vi "STAGE+mono+counter_edit-3x-error.vi"() -> ()   [LabVIEW 2017]
panel:
  out "XY Graph":cluster{"Y":dbl[], "Y":dbl[]}[](graph)
  in  "Integrating time, 10^-7 sec":dbl=10000000.0
  in  "scan from":i32=2600
  in  "scan to":i32=4000
  in  "?":bool
  in  "Exit Labview":bool
  in  "step size":dbl=10.0 min=0.0
  in  "?":bool
  out "Spectrum":waveform(dbl)(graph)
  out "Counts":i32
  in  "value (0)":dbl=-9.0
  in  "number of disc steps":i32=1
  out "Current WL Wavelength  2":u16 caption="Current Wavelength"
  out "Grt# 2":u8=1 min=1 max=3 step=1
  out "Blaze (nm)":u32=300
  out "Groove/mm":u32=1200
  in  "?":bool
  in  "Channel B Input":u16(ring)=2 items=["Input 1"=1, "Input 2"=2]
  in  "Trigger mode":u16(ring) items=["10 MHz"=0, "Input 2"=2, "Input T"=3]
  out "Current WL Wavelength":u16 caption="Current Wavelength"
  in  "Integrating time, 10^-7 sec":dbl=10000000.0
  in  "gate A mode (CW:0)":i16(slide) scale=0.0..2.0 scale format="%.2f"
  in  "Channel A Input":u16(ring)=1 items=["10 MHz", "Input 1"]
  in  "Time between measurements\n at one point (s)/Dwell Time":dbl=0.002 min=0.002 max=60.0 step=0.001
  in  "Number of Measurements\n to take at one point/ Number of Periods":u16=1 min=1 max=2000 step=1
  in  "Count Mode":u16(ring) items=["A,B for Preset T", "A-B for Preset T", "A+B for Preset T", "A for Preset B"]
  in  "GPIB address":string="23"
  out "Timeout":bool
  out "Serial":u32=12345
  out "Grt#":u8=1 min=1 max=3 step=1
  out "Blaze (nm)":u32=300
  out "Groove/mm":u32=1200
  out "time delay":u32=450000 min=1
  out "Mono port":T1(ring)
  in  "Get position":bool
  out "Position status":dbl format="%.3f"
  in  "Target position":dbl format="%.3f"
  in  "Move":bool
  in  "Motor OFF":bool
  in  "Motor ON":bool
  in  "Step Size [um]":i32=10
  in  "Axis":i32=1
  in  "Rep Rate [Hz]":dbl=500.0
  out "Shots":dbl
  in  "Averaging Time [s]":dbl=0.1
  out "Current Point":i32
  out "Slide":i32(slide) scale=0.0..100.0
  out "Current Position [mm]":dbl
  in  "Axis initial position [mm]":dbl
  out "Axis final Position [mm]":dbl
  in  "Data Points (100 default)":i32=100
  in  "Collect Data!":bool
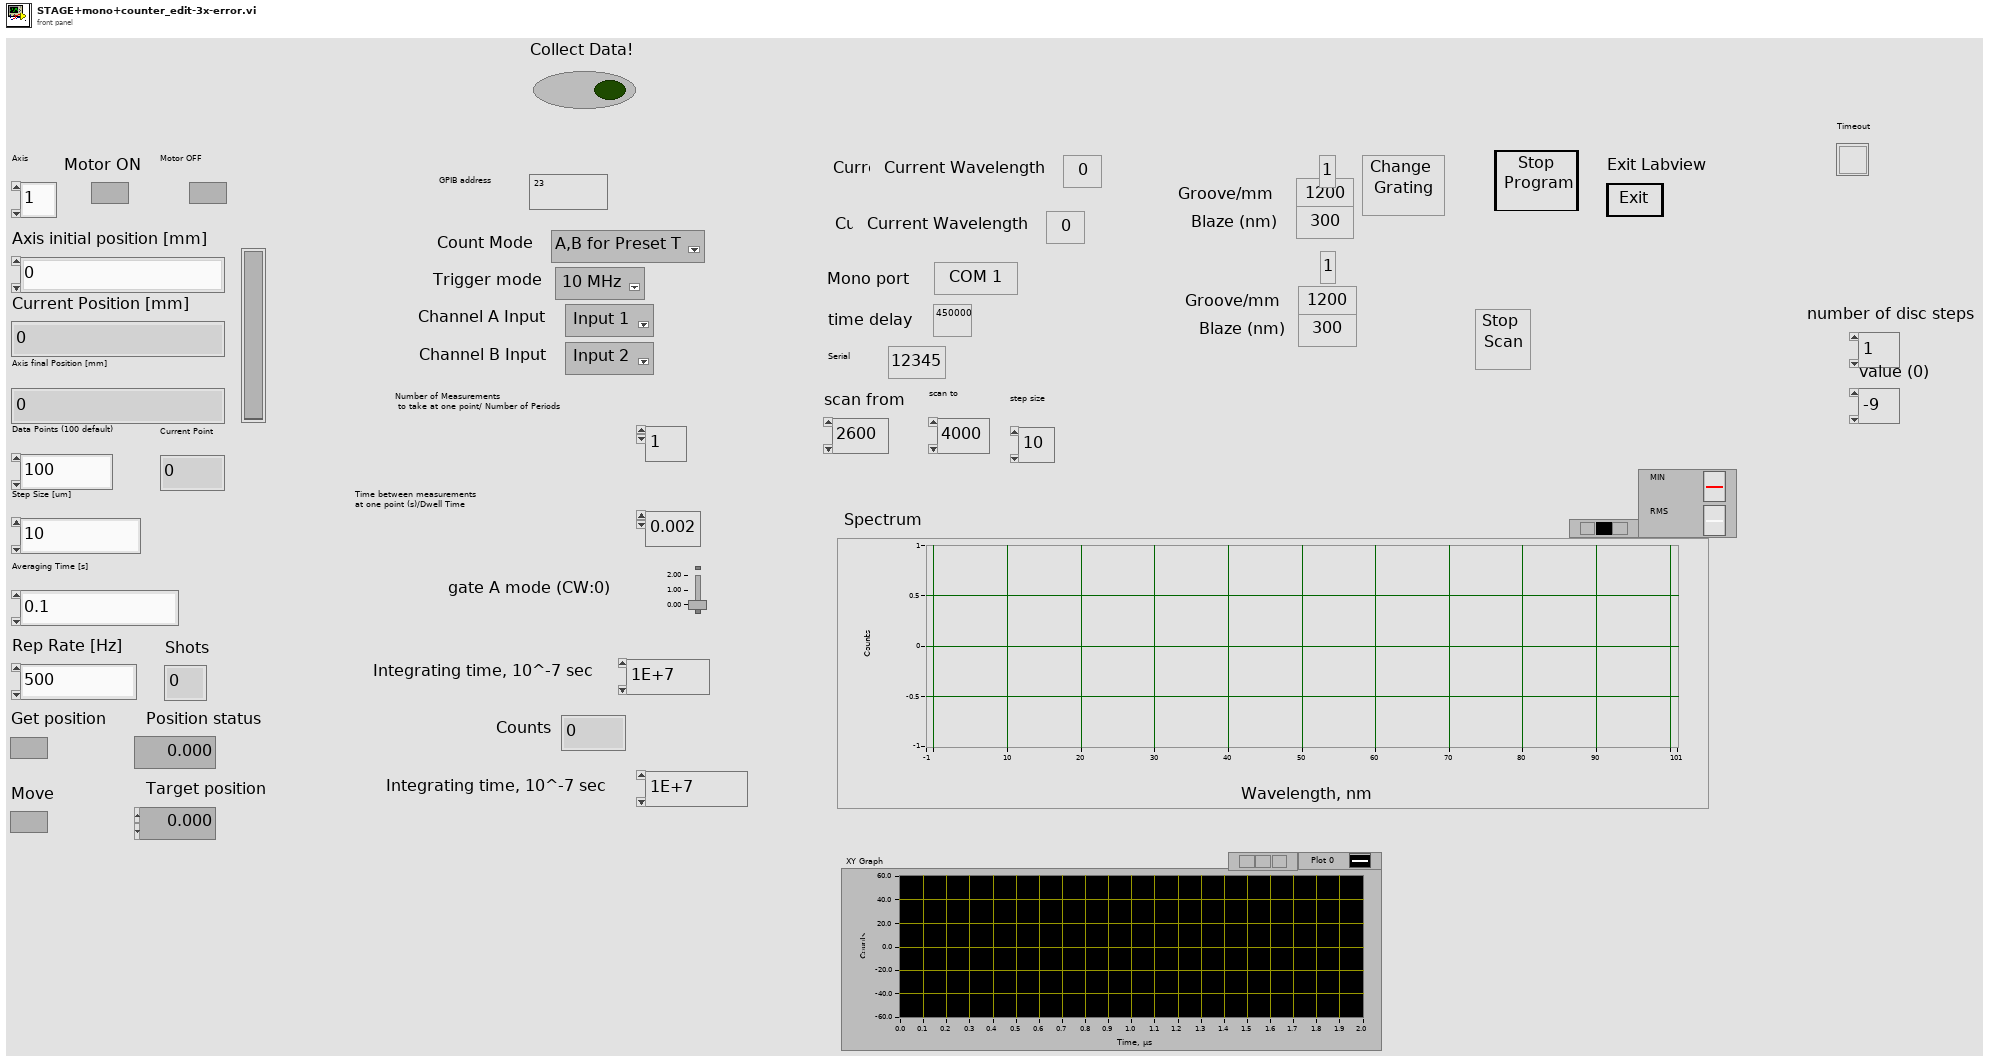
[diagram p1: front panel]
types:
  T1 = enum8{"COM 1", "COM 2", "COM 3", "COM 4", "COM 5", "COM 6", "COM 7", "COM 8", "COM 9"}
  T2 = cluster{"input XON/XOFF":bool, "input HW Handshake":bool, "input alt HW HShk":bool, "output XON/XOFF":bool, "output HW Handshake":bool, "output alt HW HShk":bool, "XOFF byte":u8, "XON byte":u8, "parity error byte":u16}
  T3 = enum16{"no parity", "odd parity", "even parity", "mark parity", "space parity"}
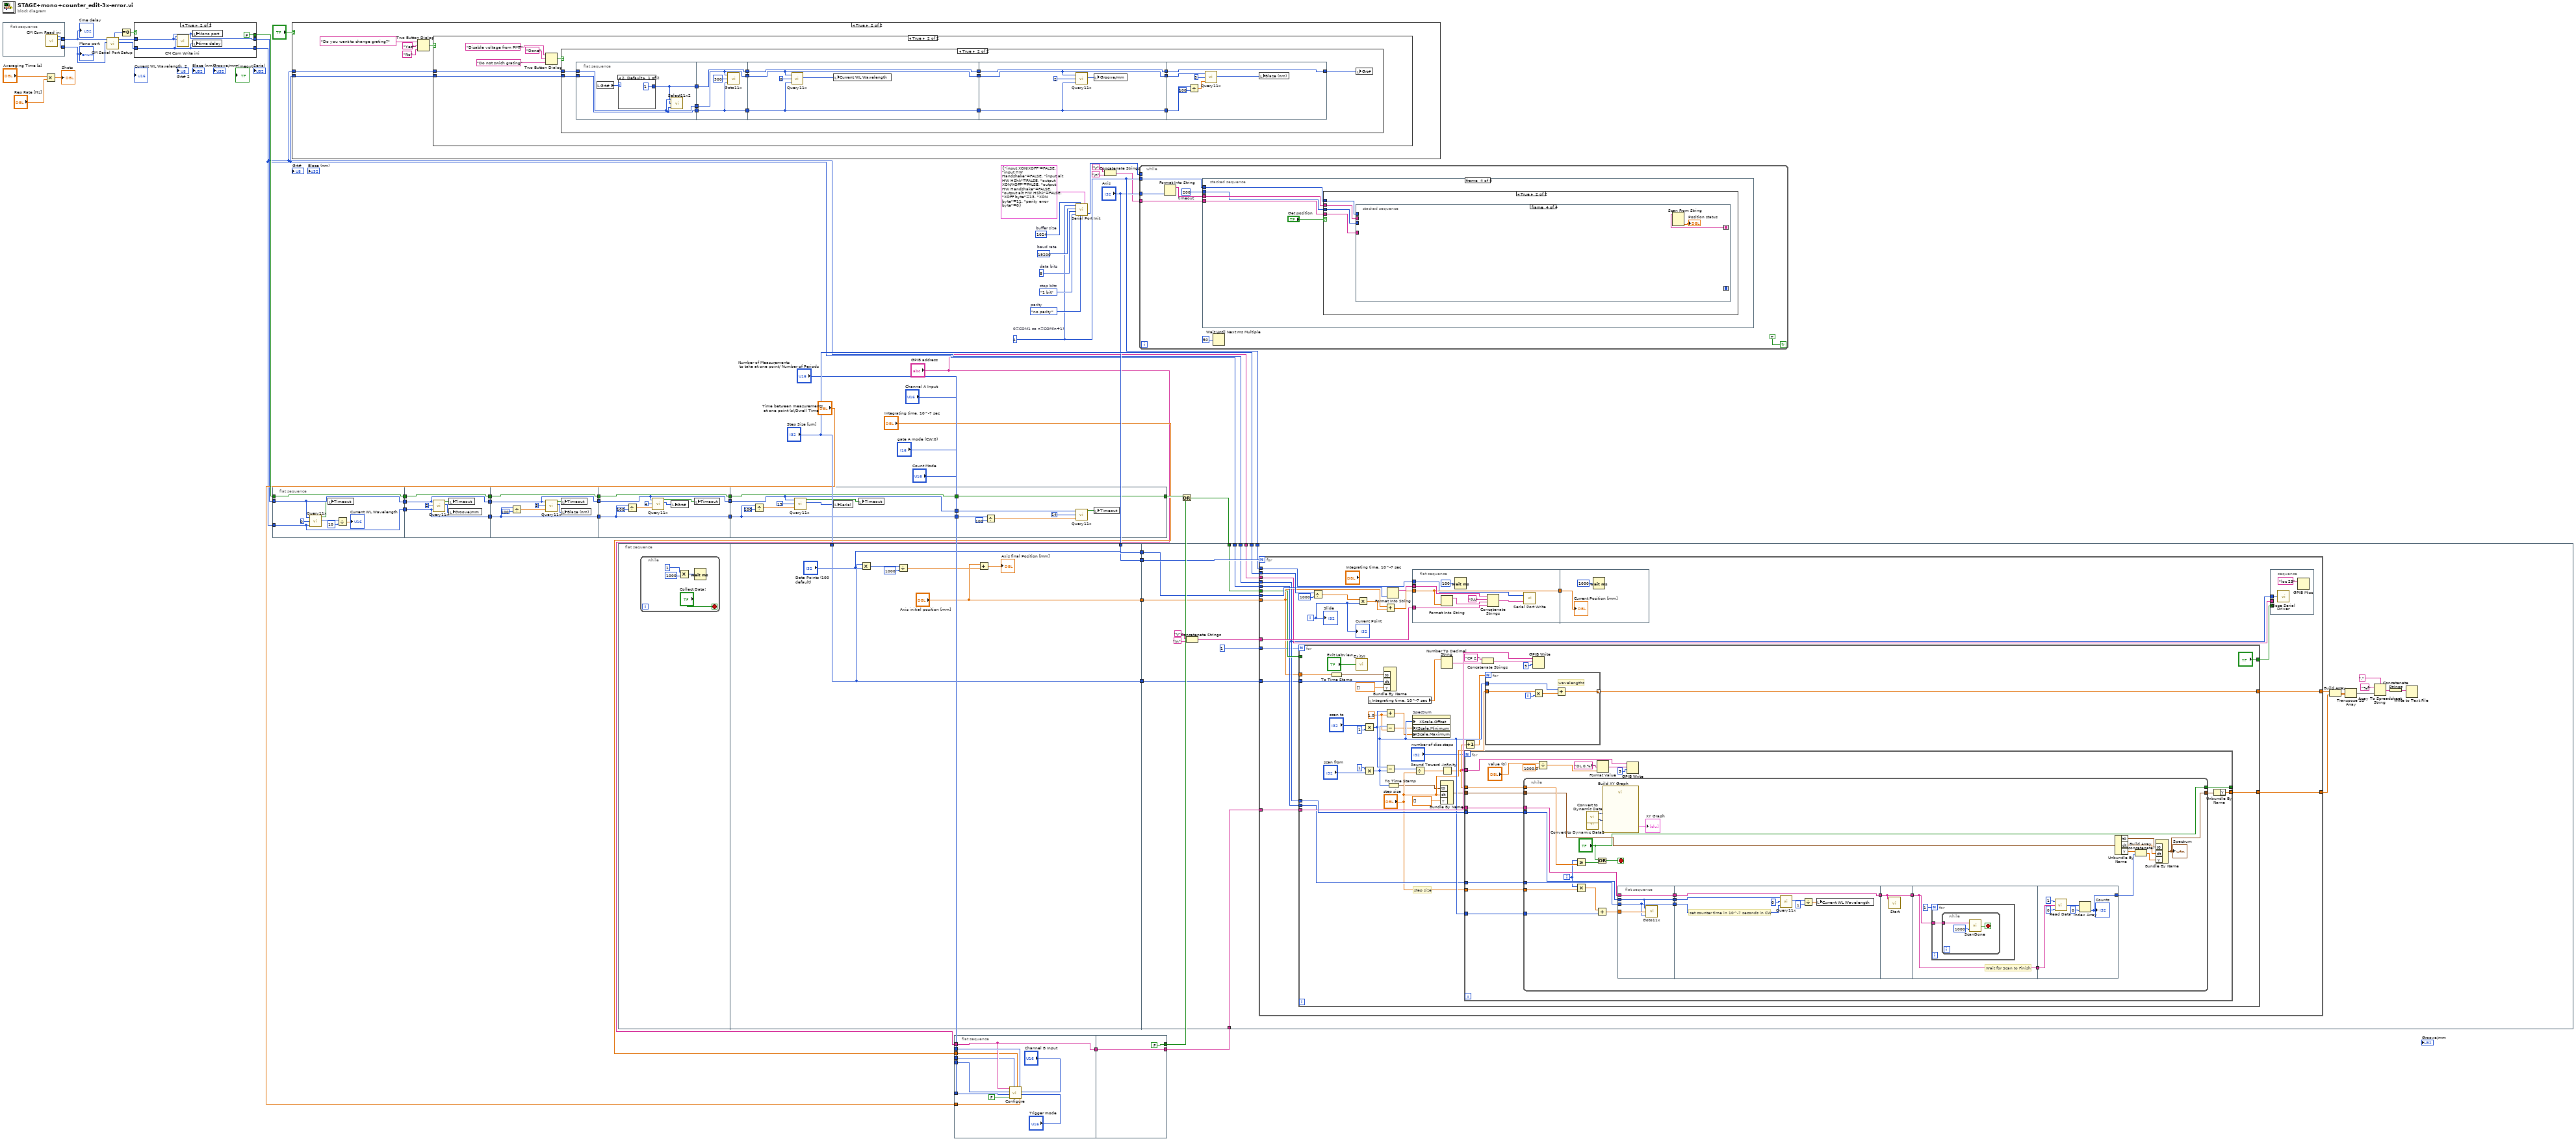
[diagram p0: block diagram]
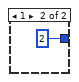
[diagram p5: hidden frame]
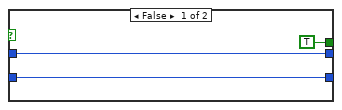
[diagram p6: hidden frame]
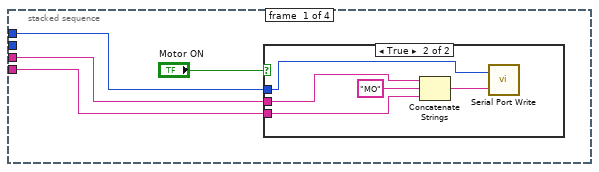
[diagram p7: hidden frame]
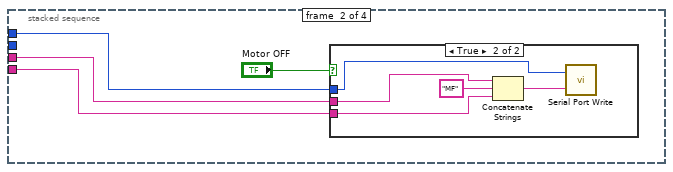
[diagram p9: hidden frame]
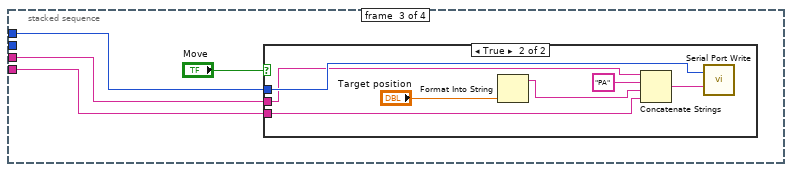
[diagram p11: hidden frame]
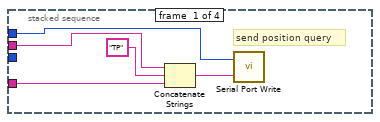
[diagram p14: hidden frame]
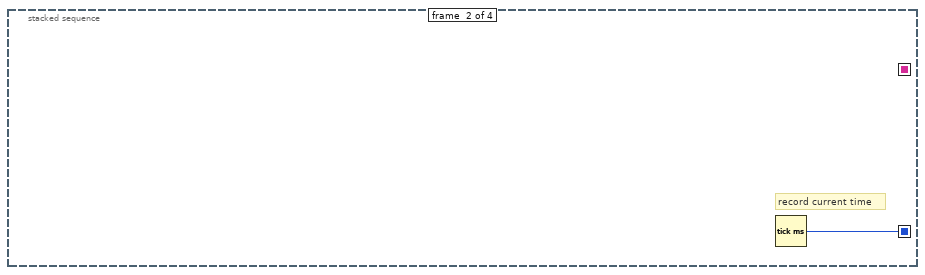
[diagram p15: hidden frame]
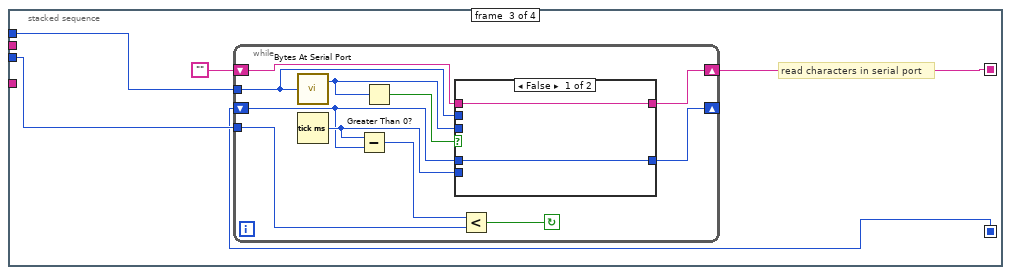
[diagram p16: hidden frame]
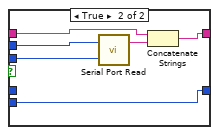
[diagram p17: hidden frame]
diagram:
  w47 = u32 19200  # baud rate
  w46 = u16 8  # data bits
  w45 = enum16{"1 bit", "1.5 bits", "2 bits"}."1 bit"  # stop bits
  w50 = T3."no parity"  # parity
  w44 = 4  # 0=COM1 so n=COM(n+1)
  w49 = u16 1024  # buffer size
  n1 = flat-sequence {
    tunnel: [w59] -> w22
    tunnel: [w58] -> w21
    frame #0 {
      n2 = call "CM Com Read ini.vi"() -> ("Mono port"=w58:T1, "time delay1"=w59:u32)  [unwired: 7 in]
    }
  }
  n3 = Multiply(x="Averaging Time [s]", y="Rep Rate [Hz]") -> (x*y=→"Shots":dbl)
  n4 = call "CM Serial Port Setup.vi"("COM port"=w21, "time delay"=w22) -> ("time delay1"=w17:u32, "DK port Out"=w18:T1, "error code"=w20:i32)  [unwired: 7 in]
  n5 = Equal To 0?(x=w20) -> (x = 0?=w19:bool)
  n6 = case shown="True" w19 {
    tunnel: w18 -> [w62 w65]
    tunnel: w17 -> [w61 w64]
    tunnel: [w62 w65] -> w4
    tunnel: [w61 w64] -> w3
    tunnel: [TRUE FALSE] -> w16
    frame False {
    }
    frame True {
      n7 = call "CM Com Write ini.vi"("time delay1"=w65, "Mono port"=w64) -> ()  [unwired: 7 in]
      n8 = local write "Mono port"(w65) -> ()
      n9 = local write "time delay"(w64) -> ()
    }
  }
  n10 = flat-sequence {
    tunnel: w3 -> [w71]
    tunnel: [w71] -> w38
    tunnel: w4 -> [w73]
    tunnel: [w73] -> w37
    tunnel: w16 -> [w69]
    tunnel: [w69] -> w36
    tunnel: w38 -> [w76]
    tunnel: [w76] -> w35
    tunnel: w37 -> [w78]
    tunnel: [w78] -> w34
    tunnel: w36 -> [w74]
    tunnel: [w74] -> w33
    tunnel: w35 -> [w86]
    tunnel: [w86] -> w32
    tunnel: w34 -> [w83]
    tunnel: [w83] -> w31
    tunnel: w33 -> [w80]
    tunnel: [w80] -> w30
    tunnel: w32 -> [w94]
    tunnel: [w94] -> w29
    tunnel: w31 -> [w91]
    tunnel: [w91] -> w28
    tunnel: w30 -> [w88]
    tunnel: [w88] -> w27
    tunnel: w29 -> [w102]
    tunnel: [w102] -> w26
    tunnel: w28 -> [w99]
    tunnel: [w99] -> w25
    tunnel: w27 -> [w96]
    tunnel: [w96] -> w24
    tunnel: w26 -> [w109]
    tunnel: w25 -> [w106]
    tunnel: [w104] -> w10
    tunnel: w24 -> [w104]
    frame #0 {
      n11 = call "Query11x.vi"("port number"=w73, "QUERY"=u16 0, "time delay"=w71) -> ("timeout"=w70:bool, "STATUS MESSAGE"=w68:u16)  [unwired: 2 out]
      n12 = local write "Timeout"(w70) -> ()
      n13 = Divide(x=w68, y=10 ("Numeric")) -> (x/y=→"Current WL Wavelength":dbl)
    }
    frame #1 {
      n14 = call "Query11x.vi"("port number"=w78, "QUERY"=u16 2, "time delay"=w76) -> ("timeout"=w75:bool, "STATUS MESSAGE"=w77:u16)  [unwired: 2 out]
      n15 = local write "Timeout"(w75) -> ()
      n16 = local write "Groove/mm"(w77) -> ()
    }
    frame #2 {
      n17 = Divide(x=w86, y=i16 100 ("device (1)")) -> (x/y=w84:dbl)
      n18 = call "Query11x.vi"("port number"=w83, "QUERY"=u16 3, "time delay"=w84) -> ("timeout"=w81:bool, "STATUS MESSAGE"=w82:u16)  [unwired: 2 out]
      n19 = local write "Timeout"(w81) -> ()
      n20 = local write "Blaze (nm)"(w82) -> ()
    }
    frame #3 {
      n21 = Divide(x=w94, y=i16 100 ("device (1)")) -> (x/y=w92:dbl)
      n22 = call "Query11x.vi"("port number"=w91, "QUERY"=u16 4, "time delay"=w92) -> ("timeout"=w89:bool, "STATUS MESSAGE"=w90:u16)  [unwired: 2 out]
      n23 = local write "Grt#"(w90) -> ()
      n24 = local write "Timeout"(w89) -> ()
    }
    frame #4 {
      n25 = Divide(x=w102, y=i16 100 ("device (1)")) -> (x/y=w100:dbl)
      n26 = call "Query11x.vi"("port number"=w99, "QUERY"=u16 19, "time delay"=w100) -> ("timeout"=w97:bool, "STATUS MESSAGE"=w98:u16)  [unwired: 2 out]
      n27 = local write "Serial"(w98) -> ()
      n28 = local write "Timeout"(w97) -> ()
    }
    frame #5 {
      n29 = Divide(x=w109, y=i16 100 ("device (1)")) -> (x/y=w107:dbl)
      n30 = call "Query11x.vi"("port number"=w106, "QUERY"=u16 14, "time delay"=w107) -> ("timeout"=w105:bool)  [unwired: 3 out]
      n31 = local write "Timeout"(w105) -> ()
    }
  }
  n32 = case shown="True" "?" {
    tunnel: w3 -> [_ w112]
    tunnel: w4 -> [_ w111]
    frame False {
    }
    frame True {
      n33 = Two Button Dialog(message="Do you want to change grating?", 1:"No" ("F button name (\"Cancel\")"), 2:"Yes" ("T button name (\"OK\")")) -> (T button?=w113:bool)
      n34 = case shown="True" w113 {
        tunnel: w112 -> [_ w118]
        tunnel: w111 -> [_ w117]
        frame False {
        }
        frame True {
          n35 = Two Button Dialog(message="Disable voltage from PMT", 1:"Do not swich grating" ("F button name (\"Cancel\")"), 2:"Done" ("T button name (\"OK\")")) -> (T button?=w119:bool)
          n36 = case shown="True" w119 {
            tunnel: w118 -> [_ w137]
            tunnel: w117 -> [_ w136]
            frame False {
            }
            frame True {
              n37 = flat-sequence {
                tunnel: w137 -> [w141]
                tunnel: [w141] -> w134
                tunnel: w136 -> [w140]
                tunnel: [w140] -> w133
                tunnel: [w138] -> w132
                tunnel: w134 -> [w145]
                tunnel: [w145] -> w131
                tunnel: w133 -> [w146]
                tunnel: [w146] -> w130
                tunnel: w132 -> [w144]
                tunnel: [w144] -> w129
                tunnel: w131 -> [w152]
                tunnel: [w152] -> w128
                tunnel: w130 -> [w151]
                tunnel: [w151] -> w127
                tunnel: w129 -> [w148]
                tunnel: [w148] -> w126
                tunnel: w128 -> [w155]
                tunnel: [w155] -> w125
                tunnel: w127 -> [w156]
                tunnel: [w156] -> w124
                tunnel: w126 -> [w153]
                tunnel: [w153] -> w123
                tunnel: w125 -> [w160]
                tunnel: w124 -> [w161]
                tunnel: [w158] -> w135
                tunnel: w123 -> [w158]
                frame #0 {
                  n38 = local read "Grt#"() -> (w139:u8)
                  n39 = case shown="2, Default" w139 {
                    tunnel: [1 2] -> w138
                    frame 2, Default {
                    }
                    frame 1 {
                    }
                  }
                  n40 = call "Select11x2.vi"("time delay"=w141, "NEW GRT?"=w138, "port number"=w140) -> ()  [unwired: 3 out]
                }
                frame #1 {
                  n41 = call "Goto11x.vi"("time delay"=w145, "WAVELENGTH"=u16 300, "port number"=w146) -> ()  [unwired: 3 out]
                }
                frame #2 {
                  n42 = call "Query11x.vi"("port number"=w151, "QUERY"=u16 0, "time delay"=w152) -> ("STATUS MESSAGE"=w149:u16)  [unwired: 3 out]
                  n43 = local write "Current WL Wavelength"(w149) -> ()
                }
                frame #3 {
                  n44 = call "Query11x.vi"("port number"=w156, "QUERY"=u16 2, "time delay"=w155) -> ("STATUS MESSAGE"=w154:u16)  [unwired: 3 out]
                  n45 = local write "Groove/mm"(w154) -> ()
                }
                frame #4 {
                  n46 = Divide(x=w160, y=i16 100 ("device (1)")) -> (x/y=w162:dbl)
                  n47 = call "Query11x.vi"("port number"=w161, "QUERY"=u16 3, "time delay"=w162) -> ("STATUS MESSAGE"=w159:u16)  [unwired: 3 out]
                  n48 = local write "Blaze (nm)"(w159) -> ()
                }
              }
              n49 = local write "Grt#"(w135) -> ()
            }
          }
        }
      }
    }
  }
  n50 = flat-sequence {
    tunnel: ["Data Points (100 default)"] -> w57
    tunnel: "Axis" -> [w176]
    tunnel: ["Axis initial position [mm]"] -> w56
    tunnel: "Step Size [um]" -> [w169]
    tunnel: [w176] -> w55
    tunnel: [w169] -> w1
    tunnel: w57 -> [w199]
    tunnel: w56 -> [w198]
    tunnel: "Step Size [um]" -> [w197]
    tunnel: w55 -> [w196]
    tunnel: w44 -> [w192]
    tunnel: w6 -> [w191]
    tunnel: w5 -> [w190]
    tunnel: w4 -> [w189]
    tunnel: w3 -> [w188]
    tunnel: "GPIB address" -> [w187]
    tunnel: w1 -> [w185]
    frame #0 {
      n51 = while {
        stop <- "Collect Data!" stop-if-true
        n52 = Multiply(x=1, y=1000) -> (x*y=w168:i32)
        n53 = Wait (ms)(milliseconds to wait=w168) -> ()  [unwired: 1 out]
      }
    }
    frame #1 {
      n54 = Multiply(x=w169, y="Data Points (100 default)") -> (x*y=w172:i32)
      n55 = Divide(x=w172, y=1000) -> (x/y=w171:dbl)
      n56 = Add(x="Axis initial position [mm]", y=w171) -> (x+y=→"Axis final Position [mm]":dbl)
    }
    frame #2 {
      n57 = Concatenate Strings("\r", "\n") -> (w193:string)
      n58 = for {
        N: w199 -> [_]
        tunnel: w198 -> [w203]
        tunnel: w197 -> [w217]
        tunnel: w196 -> [w214]
        tunnel: w193 -> [w211]
        tunnel: w192 -> [w212]
        tunnel: w191 -> [w209]
        tunnel: w190 -> [w208]
        tunnel: w189 -> [w205]
        tunnel: w188 -> [w207]
        tunnel: w187 -> [w206]
        tunnel: 1 -> [w204]
        tunnel: w185 -> [w202]
        tunnel: [w201] -> w180
        tunnel: [w200] -> w179
        i -> [w221]
        n59 = for {
          N: w204 -> [_]
          tunnel: w205 -> [w252]
          tunnel: w207 -> [w244]
          tunnel: ["?"] -> w210
          tunnel: w208 -> [_]
          tunnel: w209 -> [w251]
          tunnel: w203 -> [w243]
          tunnel: w202 -> [w242]
          tunnel: [w223] -> w201
          tunnel: [w222] -> w200
          w239 = 1.0 ("x")
          # "step size"
          n60 = To Time Stamp(1:w243) -> (0:w225:timestamp)
          n61 = call "ExitVI.vi"("Exit Labview"="Exit Labview") -> ()
          n62 = Multiply(x="scan to", y=1) -> (x*y=w248:i32)
          n63 = Multiply(x=1, y="scan from") -> (x*y=w246:i32)
          n64 = local read "Integrating time, 10^-7 sec"() -> (w235:dbl)
          n65 = Bundle By Name("t0"=w225, "dt"=w242, "Y"=dbl[] []) -> ()  [unwired: 1 in, 1 out]
          n66 = Add(x=w248, y=w239) -> (x+y=w240:dbl)
          n67 = Subtract(x=w246, y=w239) -> (x-y=w238:dbl)
          n68 = Subtract(x=w248, y=w246) -> (x-y=w255:i32)
          n69 = To Time Stamp(1:w246) -> (0:w233:timestamp)
          n70 = property on="Spectrum" class="WFGraph (strict)"("XScale.Offset"=w246, "XScale.Minimum"=w238, "XScale.Maximum"=w240) -> ()  [unwired: 2 in, 2 out]
          n71 = Divide(x=w255, y="step size") -> (x/y=w241:dbl)
          n72 = Bundle By Name("t0"=w233, "dt"="step size", "Y"=dbl[] []) -> (w232:waveform(dbl))  [unwired: 1 in]
          n73 = Number To Decimal String(number=w235) -> (decimal integer string=w229:string)  [unwired: 1 in]
          n74 = Round Toward -Infinity(1:w241) -> (0:w236:dbl)
          n75 = Increment(x=w236) -> (x+1=w231:dbl)
          n76 = for {
            N: "number of disc steps" -> [_]
            tunnel: "step size" -> [w272]
            tunnel: w252 -> [w271]
            tunnel: w244 -> [w270]
            tunnel: w236 -> [w269]
            tunnel: w232 -> [w268]
            tunnel: [w267] -> _
            tunnel: w246 -> [w266]
            tunnel: w251 -> [w265]
            tunnel: [w263] -> w222
            tunnel: w251 -> [w259]
            n77 = while {
              tunnel: w266 -> [w288]
              tunnel: w272 -> [w300]
              tunnel: w271 -> [w298]
              tunnel: w270 -> [w297]
              tunnel: w269 -> [w296]
              tunnel: ["?"] -> w267
              tunnel: w265 -> [w283]
              tunnel: w268 -> [w294]
              tunnel: [w284] -> w264
              i -> [w291]
              stop <- w295 stop-if-true
              n78 = Greater Or Equal?(x=w291, y=w296) -> (x >= y?=w285:bool)
              n79 = Multiply(x=w291, y=w300) -> (x*y=w299:dbl)
              n80 = call "Convert to Dynamic Data"() -> ("Dynamic Data Type"=w275:dynamicdata)  [unwired: 4 in]
              n81 = call "Convert to Dynamic Data2"() -> ("Dynamic Data Type"=w274:dynamicdata)  [unwired: 4 in]
              n82 = Or(x="?", y=w285) -> (x .or. y?=w295:bool)
              n83 = Add(x=w299, y=w288) -> (x+y=w287:dbl)
              n84 = call "Build XY Graph"("Y Input"=w274, "X Input"=w275) -> ("XY Graph"=→"XY Graph":cluster{"Y":dbl[], "Y":dbl[]}[])  [unwired: 3 in, 6 out]
              n85 = flat-sequence {
                tunnel: w287 -> [w304]
                tunnel: w298 -> [w303]
                tunnel: [w303] -> w281
                tunnel: w297 -> [w302]
                tunnel: [w302] -> w280
                tunnel: w283 -> [w301]
                tunnel: [w301] -> w279
                tunnel: w281 -> [w310]
                tunnel: w280 -> [w309]
                tunnel: w279 -> [w308]
                tunnel: [w308] -> w278
                tunnel: w278 -> [w312]
                tunnel: [w312] -> w277
                tunnel: w277 -> [w313]
                tunnel: [w313] -> w276
                tunnel: w276 -> [w320]
                tunnel: [w319] -> w282
                frame #0 {
                  n86 = call "Goto11x.vi"("time delay"=w302, "WAVELENGTH"=w304, "port number"=w303) -> ()  [unwired: 3 out]
                }
                frame #1 {
                  # "set counter time in 10^-7 seconds in CW"
                  n87 = call "Query11x.vi"("port number"=w310, "QUERY"=0, "time delay"=w309) -> ("STATUS MESSAGE"=w307:u16)  [unwired: 3 out]
                  n88 = Divide(x=w307, y=1) -> (x/y=w306:dbl)
                  n89 = local write "Current WL Wavelength"(w306) -> ()
                }
                frame #2 {
                  n90 = call "Start.vi"("GPIB Address"=w312) -> ()  [unwired: 9 in]
                }
                frame #3 {
                  # "Wait for Scan to Finish"
                  n91 = for {
                    N: 1 -> [_]
                    tunnel: w313 -> [w315]
                    n92 = while {
                      tunnel: w315 -> [w316]
                      stop <- w318 stop-if-true
                      n93 = call "ScanDone.vi"("Wait (ms)"=1000, "GPIB Address"=w316) -> ("Scan Finished?"=w318:bool)
                    }
                  }
                }
                frame #4 {
                  n94 = call "Read Data.vi"("Channel Number"=0, "GPIB Address"=w320, "Number of Datapoints"=1) -> ("Data"=w321:i32[])
                  n95 = Index Array(array=w321, index=0) -> (element=w319:i32)
                  "Counts" <- w319
                }
              }
              n96 = Unbundle By Name(w294) -> ("t0"=w292:timestamp, "dt"=w293:dbl, "Y"=w290:dbl[])
              n97 = Build Array (concatenate)(w290, w282) -> (w289:dbl[])
              n98 = Bundle By Name("t0"=w292, "dt"=w293, "Y"=w289) -> (w284:waveform(dbl))  [unwired: 1 in]
              "Spectrum" <- w284
            }
            n99 = Divide(x="value (0)", y=1000.0) -> (x/y=w256:dbl)
            n100 = Format Value(format string="DL 0,%f;", value (0)=w256) -> (output string=w261:string)  [unwired: 1 in]
            n101 = GPIB Write(0:w259, 1:w261, 2:i16 5 ("mode (0)")) -> ()  [unwired: 2 in, 2 out]
            n102 = Unbundle By Name(w264) -> ("Y"=w263:dbl[])
          }
          n103 = Concatenate Strings("CP 2,", w229) -> (w227:string)
          n104 = for {
            N: w231 -> [_]
            tunnel: "step size" -> [w329]
            tunnel: w246 -> [w327]
            tunnel: [w325] -> w223 mode=indexing
            i -> [w328]
            # "wavelengths"
            n105 = Multiply(x=w329, y=w328) -> (x*y=w326:dbl)
            n106 = Add(x=w327, y=w326) -> (x+y=w325:dbl)
          }
          n107 = GPIB Write(0:w251, 1:w227, 2:i16 5 ("mode (0)")) -> ()  [unwired: 2 in, 2 out]
        }
        n108 = Divide(x=w217, y=1000) -> (x/y=w216:dbl)
        n109 = Multiply(x=w216, y=w221) -> (x*y=w220:dbl)
        n110 = Add(x=w203, y=w220) -> (x+y=w219:dbl)
        n111 = Format Into String(w214) -> (resulting string=w213:string)  [unwired: 3 in, 1 out]
        n112 = flat-sequence {
          tunnel: w219 -> [w334]
          tunnel: [w334] -> w215
          tunnel: w211 -> [w336]
          tunnel: w213 -> [w335]
          tunnel: w212 -> [w332]
          tunnel: w215 -> [w340]
          frame #0 {
            n113 = Format Into String(w334) -> (resulting string=w333:string)  [unwired: 3 in, 1 out]
            n114 = Wait (ms)(milliseconds to wait=u32 100) -> ()  [unwired: 1 out]
            n115 = Concatenate Strings(w335, "PA" ("Substring"), w333, w336) -> (w338:string)
            n116 = call <vilib>:"Serial Port Write.vi"("string to write"=w338, "port number"=w332) -> ()  [unwired: 1 out]
          }
          frame #1 {
            n117 = Wait (ms)(milliseconds to wait=u32 1000) -> ()  [unwired: 1 out]
            "Current Position [mm]" <- w340
          }
        }
        n118 = stacked-sequence {
          tunnel: w210 -> [_]
          tunnel: w205 -> [w331]
          tunnel: w206 -> [_]
          frame #0 {
            n119 = call <vilib>:"Close Serial Driver.vi"("port number"=w331) -> ()  [unwired: 1 out]
            n120 = GPIB Misc(0:"loc 23" ("command string")) -> ()  [unwired: 1 in, 3 out]
          }
        }
        "Current Point" <- w221
        "Slide" <- w221
      }
      n121 = Build Array(w180, w179) -> (w182:dbl[][])
      n122 = Transpose 2D Array(2D array=w182) -> (transposed array=w181:dbl[][])
      n123 = Array To Spreadsheet String(delimiter (Tab)=",", array=w181, 3:"%f" ("format string")) -> (spreadsheet string=w183:string)
      n124 = Concatenate Strings(w183) -> (w184:string)
      n125 = Write to Text File(text=w184) -> ()  [unwired: 3 in, 3 out]
    }
  }
  n126 = flat-sequence {
    tunnel: "GPIB address" -> [w349]
    tunnel: [w349] -> w23
    tunnel: "Count Mode" -> [w350]
    tunnel: "Number of Measurements\n to take at one point/ Number of Periods" -> [w347]
    tunnel: "Time between measurements\n at one point (s)/Dwell Time" -> [w346]
    tunnel: "Channel A Input" -> [w351]
    tunnel: "gate A mode (CW:0)" -> [w343]
    tunnel: "Integrating time, 10^-7 sec" -> [w342]
    tunnel: w23 -> [w352]
    tunnel: [w352] -> w6
    tunnel: [FALSE] -> w11
    frame #0 {
      n127 = call "Configure.vi"("Dwell Time (s)"=w346, "Channel T Input"="Trigger mode", "Channel B Input"="Channel B Input", "Channel A Input"=w351, "Integrating time, 10^-7 sec"=w342, "gate mode (CW:0)"=w343, "Scan End Mode"=FALSE, "Number of Periods"=w347, "Count Mode"=w350, "GPIB Address"=w349) -> ()
    }
    frame #1 {
    }
  }
  n128 = call <vilib>:"Serial Port Init.vi"("flow control etc."=T2 {"input XON/XOFF"=FALSE, "input HW Handshake"=FALSE, "input alt HW HShk"=FALSE, "output XON/XOFF"=FALSE, "output HW Handshake"=FALSE, "output alt HW HShk"=FALSE, "XOFF byte"=13, "XON byte"=11, "parity error byte"=0}, "parity"=w50, "buffer size"=w49, "stop bits"=w45, "data bits"=w46, "baud rate"=w47, "port number"=w44) -> ("error code"=w43:i32)
  n129 = Concatenate Strings("\r", "\n") -> (w39:string)
  n130 = while {
    tunnel: w44 -> [w356]
    tunnel: w39 -> [w357]
    tunnel: w43 -> [_]
    tunnel: "Axis" -> [w354]
    stop <- TRUE continue-if-true
    w355 = u32 200  # timeout
    n131 = Format Into String(w354) -> (resulting string=w358:string)  [unwired: 3 in, 1 out]
    n132 = stacked-sequence {
      tunnel: w358 -> [w362 w372 w381 w393]
      tunnel: w357 -> [w361 w371 w380 w390]
      tunnel: w356 -> [w363 w373 w382 w392]
      tunnel: w355 -> [_ _ _ w391]
      frame #0 {
        n133 = case shown="True" "Motor ON" {
          tunnel: w363 -> [_ w369]
          tunnel: w362 -> [_ w366]
          tunnel: w361 -> [_ w365]
          frame False {
          }
          frame True {
            n134 = Concatenate Strings(w366, "MO" ("Substring"), w365) -> (w367:string)
            n135 = call <vilib>:"Serial Port Write.vi"("string to write"=w367, "port number"=w369) -> ()  [unwired: 1 out]
          }
        }
      }
      frame #1 {
        n136 = case shown="True" "Motor OFF" {
          tunnel: w373 -> [_ w378]
          tunnel: w372 -> [_ w375]
          tunnel: w371 -> [_ w374]
          frame False {
          }
          frame True {
            n137 = Concatenate Strings(w375, "MF" ("Substring"), w374) -> (w376:string)
            n138 = call <vilib>:"Serial Port Write.vi"("string to write"=w376, "port number"=w378) -> ()  [unwired: 1 out]
          }
        }
      }
      frame #2 {
        n139 = case shown="True" "Move" {
          tunnel: w382 -> [_ w389]
          tunnel: w381 -> [_ w386]
          tunnel: w380 -> [_ w385]
          frame False {
          }
          frame True {
            n140 = Format Into String("Target position") -> (resulting string=w383:string)  [unwired: 3 in, 1 out]
            n141 = Concatenate Strings(w386, "PA" ("Substring"), w383, w385) -> (w387:string)
            n142 = call <vilib>:"Serial Port Write.vi"("string to write"=w387, "port number"=w389) -> ()  [unwired: 1 out]
          }
        }
      }
      frame #3 {
        n143 = case shown="True" "Get position" {
          tunnel: w393 -> [_ w398]
          tunnel: w392 -> [_ w397]
          tunnel: w391 -> [_ w396]
          tunnel: w390 -> [_ w395]
          frame False {
          }
          frame True {
            n144 = stacked-sequence {
              seq-local: [_ w404 _ _] -> [_ _ w406 _]
              seq-local: [_ _ w405 _] -> [_ _ _ w430]
              tunnel: w398 -> [w401 _ _ _]
              tunnel: w397 -> [w400 _ w409 _]
              tunnel: w396 -> [_ _ w407 _]
              tunnel: w395 -> [w399 _ _ _]
              frame #0 {
                # "send position query"
                n145 = Concatenate Strings(w401, "TP" ("Substring"), w399) -> (w402:string)
                n146 = call <vilib>:"Serial Port Write.vi"("string to write"=w402, "port number"=w400) -> ()  [unwired: 1 out]
              }
              frame #1 {
                # "record current time"
                n147 = Tick Count (ms)() -> (millisecond timer value=w404:u32)
              }
              frame #2 {
                # "read characters in serial port"
                n148 = while {
                  shift-left: w406 -> [w410]
                  shift-right: [w411] -> _
                  tunnel: w407 -> [w414]
                  shift-left: "" -> [w417]
                  shift-right: [w416] -> w405
                  tunnel: w409 -> [w418]
                  stop <- w413 continue-if-true
                  n149 = call <vilib>:"Bytes At Serial Port.vi"("port number"=w418) -> ("byte count"=w419:u32)  [unwired: 1 out]
                  n150 = Tick Count (ms)() -> (millisecond timer value=w412:u32)
                  n151 = Subtract(x=w412, y=w410) -> (x-y=w415:u32)
                  n152 = Greater Than 0?(x=w419) -> (x > 0?=w420:bool)
                  n153 = case shown="False" w420 {
                    tunnel: w419 -> [_ w428]
                    tunnel: w418 -> [_ w427]
                    tunnel: w417 -> [w422 w425]
                    tunnel: [w422 w424] -> w416
                    tunnel: [w421 w423] -> w411
                    tunnel: w412 -> [_ w423]
                    tunnel: w410 -> [w421 _]
                    frame False {
                    }
                    frame True {
                      n154 = call <vilib>:"Serial Port Read.vi"("requested byte count"=w428, "port number"=w427) -> ("string read"=w426:string)  [unwired: 1 out]
                      n155 = Concatenate Strings(w425, w426) -> (w424:string)
                    }
                  }
                  n156 = Less?(x=w415, y=w414) -> (x < y?=w413:bool)
                }
              }
              frame #3 {
                n157 = Scan From String(input string=w430) -> (output 1=→"Position status":dbl)  [unwired: 4 in, 3 out]
              }
            }
          }
        }
      }
    }
    n158 = Wait Until Next ms Multiple(millisecond multiple=u32 50) -> ()  [unwired: 1 out]
  }
  n159 = Or(x=w10, y=w11) -> (x .or. y?=w5:bool)
  "Mono port" <- w21
  "time delay" <- w22
